vi "Kinect Basic Recorder.vi"() -> ()   [LabVIEW 2011]
uses:
  <vilib>/Utility/sysdir.llb/System Directory Type.ctl
  <vilib>/vision/NI_Vision_Development_Module.lvlib
panel:
  in  "Contour Length Threshold":dbl(slide)=126.92307692307692 min=-32768.0 max=32768.0 step=1.0 scale=0.0..500.0
  in  "Display Type":T1(ring)=enum."Baseline Extracted"
  in  "Post Extraction Limit":cluster{dbl, dbl}(slide)={48.0, 888.0} scale=-3000.0..3000.0
  in  "stop 2":bool
  in  "# Frames in Average":i32=100
  in  "Start":bool
  in  "Zero Out Baseline":bool
  in  "Median Filter Size":i32=5 min=0 max=7
  in  "Divisor":sgl=0.5 min=0 max=1 step=0.1
  in  "Name or Relative Path":string="Mouse Test"
  in  "Distance to Camera Visible":cluster{dbl, dbl}(slide)={-4718.592, 13369.344000000001} scale=-32768.0..32768.0
  in  "Status":string
  out "Frame Display":T2(plugin-control)
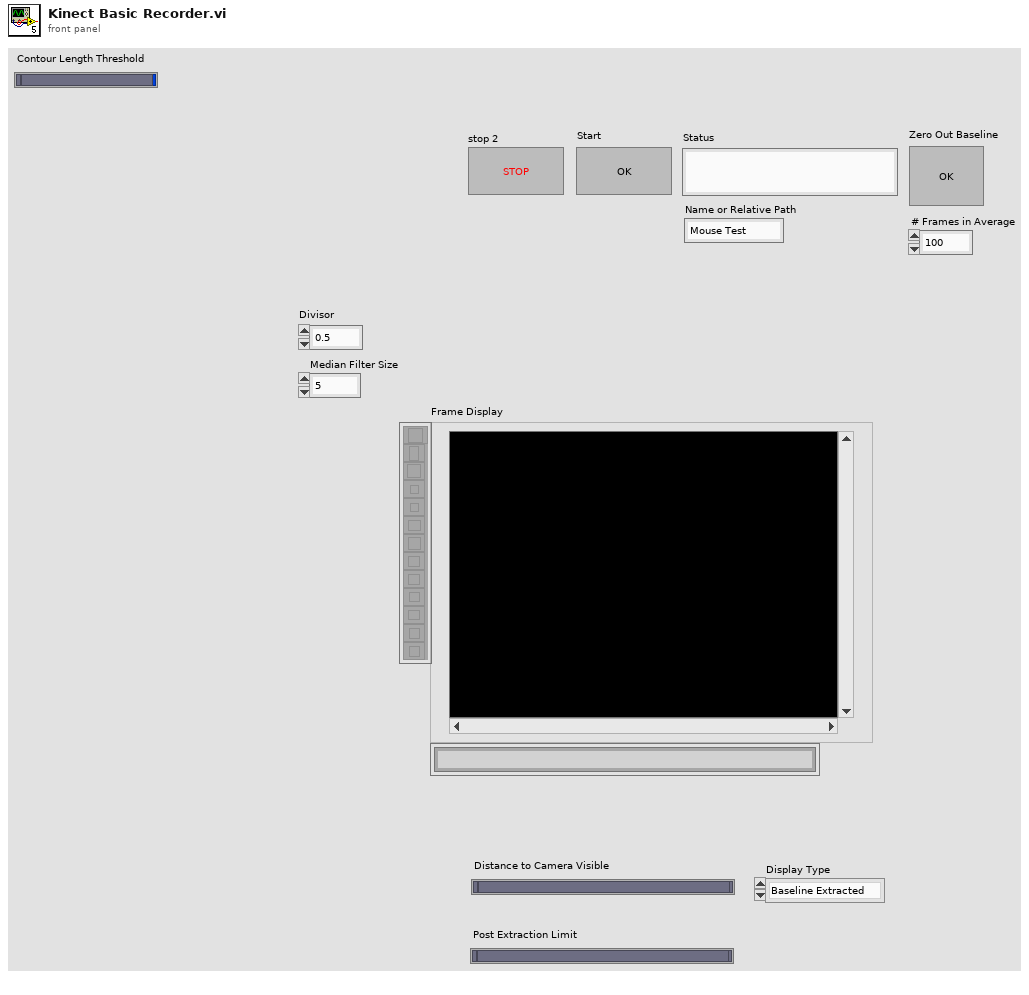
[diagram p1: front panel]
types:
  T1 = enum16{"Raw Image", "Baseline", "Baseline Extracted"}
  T2 = typedef "IMAQ Image.ctl" = refnum<image>
  T3 = typedef "System Directory Type.ctl" = i32
  T4 = enum16{"Record", "Idle", "Acquire Background", "Stop"}
  T5 = enum32{"Average", "Min", "Max", "Clear  if < ", "Clear  if < or =", "Clear  if =", "Clear  if > or =", "Clear  if >"}
  T6 = typedef "Image Type" = u32
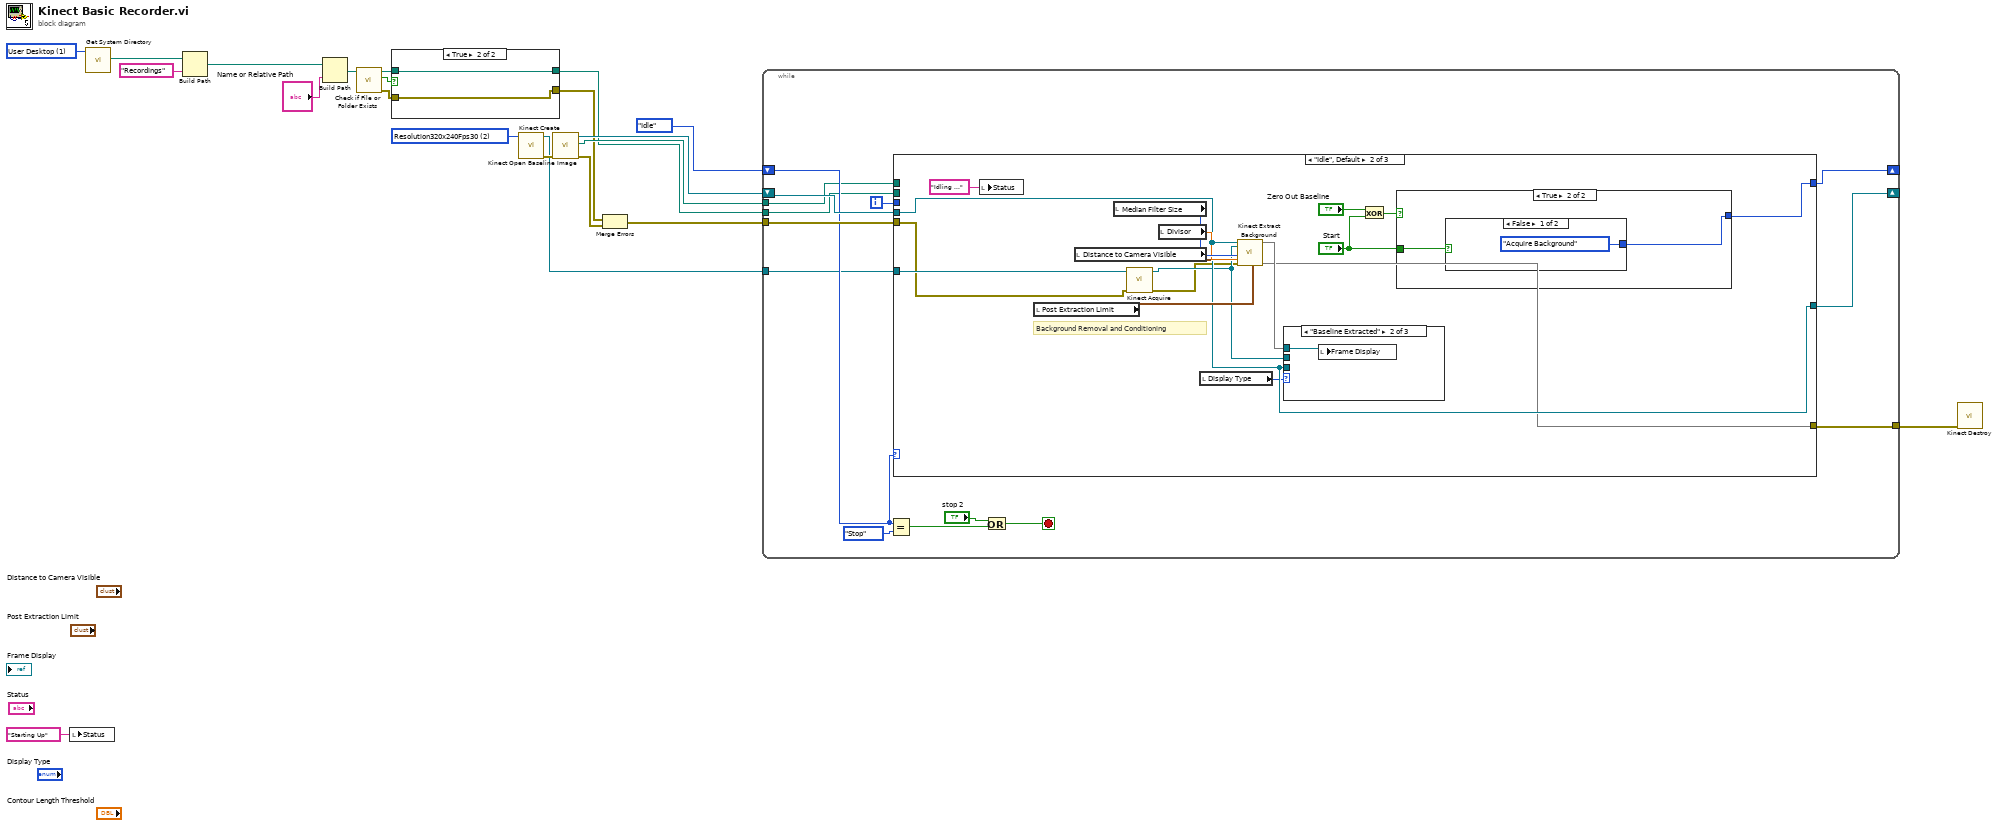
[diagram p0: block diagram]
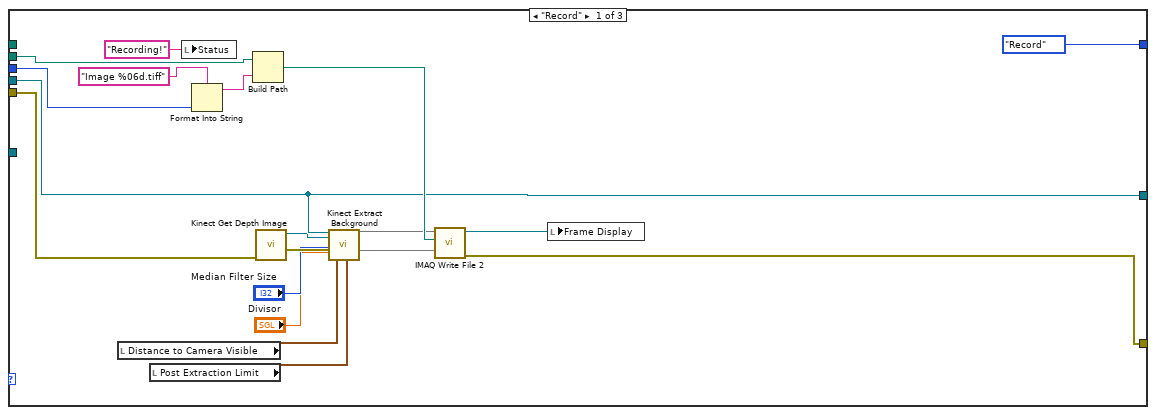
[diagram p2: hidden frame]
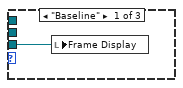
[diagram p3: hidden frame]
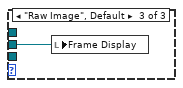
[diagram p4: hidden frame]
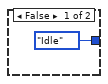
[diagram p5: hidden frame]
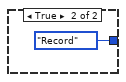
[diagram p6: hidden frame]
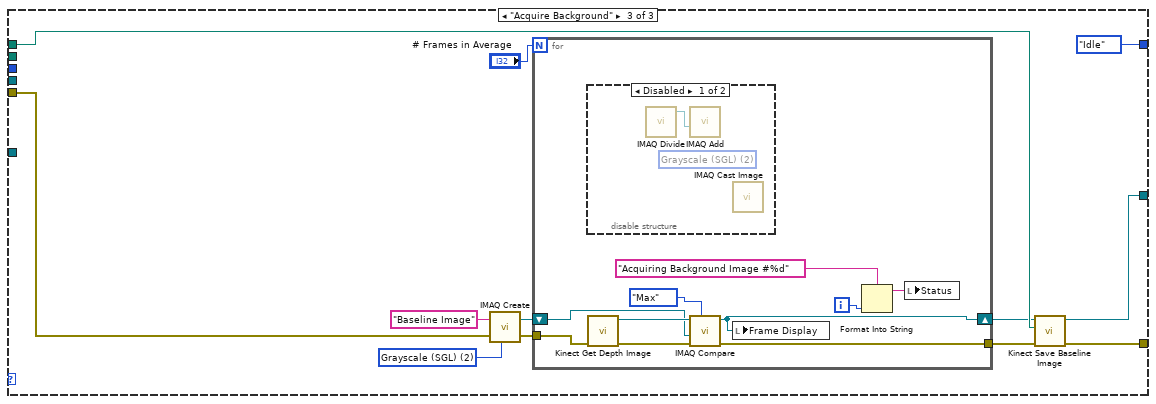
[diagram p7: hidden frame]
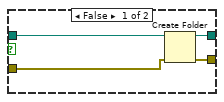
[diagram p9: hidden frame]
diagram:
  w17 = 2 items=["Undefined", "Resolution640x480Fps30", "Resolution320x240Fps30", "Resolution80x60Fps30"] ("Depth Format")
  w19 = T3 1 items=["User Home"=0, "User Desktop"=1, "User Documents"=2, "User Application Data"=3, "User Preferences"=4, "User Temporary"=5, "Public Documents"=6, "Public Application Data"=7, "Public Preferences"=8, "Public Cache"=13, "System Core Libraries"=9, "System Installed Libraries"=10, "Application Files"=11, "Boot Volume Root"=12] ("system directory type")
  n1 = local write "Status"("Starting Up" ("Status")) -> ()
  n2 = call <vilib>:"Get System Directory.vi"("system directory type"=w19) -> ("system directory"=w18:path)  [unwired: 10 in]
  n3 = Build Path(base path=w18, name or relative path="Recordings") -> (appended path=w12:path)
  n4 = Build Path(base path=w12, name or relative path="Name or Relative Path") -> (appended path=w3:path)
  n5 = call <vilib>:"Check if File or Folder Exists.vi"("path"=w3) -> ("error out"=w10:errorcluster, "file or folder exists?"=w8:bool, "dup path"=w9:path)  [unwired: 8 in]
  n6 = case shown="True" w8 {
    tunnel: w10 -> [w25 w26]
    tunnel: w9 -> [w24 w27]
    tunnel: [w22 w27] -> w7
    tunnel: [w23 w26] -> w4
    frame False {
      n7 = Create Folder(path (use dialog)=w24, error in=w25) -> (created path=w22:path, error out=w23:errorcluster)  [unwired: 1 in, 1 out]
    }
    frame True {
    }
  }
  n8 = call "Kinect Create.vi"("Depth Format"=w17) -> ("error out"=w14:errorcluster, "Kinect Acquisition Queue"=w1:refnum<queue>)  [unwired: 9 in]
  n9 = call "Kinect Open Baseline Image.vi"("error in (no error)"=w14) -> ("error out"=w5:errorcluster, "Background Image Path"=w15:path, "Background Image"=w16:T2)  [unwired: 8 in]
  n10 = Merge Errors(w4, w5) -> (w6:errorcluster)
  n11 = while {
    tunnel: w6 -> [w41]
    tunnel: [w40] -> w2
    shift-right: [w33] -> _
    shift-left: T4."Idle" -> [w35]
    shift-right: [w32] -> _
    shift-left: w16 -> [w39]
    tunnel: w15 -> [w31]
    tunnel: w7 -> [w29]
    tunnel: w1 -> [w28]
    i -> [w30]
    stop <- w37 stop-if-true
    n12 = Equal?(x=w35, y=T4."Stop") -> (x = y?=w36:bool)
    n13 = case shown="\"Idle\", Default" w35 {
      tunnel: w41 -> [w53 w62 w93]
      tunnel: [w42 w65 w89] -> w40
      tunnel: w39 -> [w51 w68 _]
      tunnel: [T4."Record" w73 T4."Idle"] -> w33
      tunnel: [w51 w68 w90] -> w32
      tunnel: w31 -> [_ _ w87]
      tunnel: w30 -> [w56 _ _]
      tunnel: w29 -> [w55 _ _]
      tunnel: w28 -> [_ w63 _]
      frame "Record" {
        n14 = local read "Distance to Camera Visible"() -> (w47:cluster{dbl, dbl})
        n15 = local read "Post Extraction Limit"() -> (w46:cluster{dbl, dbl})
        n16 = local write "Status"("Recording!" ("Status")) -> ()
        n17 = Format Into String(format string="Image %06d.tiff", w56) -> (resulting string=w57:string)  [unwired: 2 in, 1 out]
        n18 = Build Path(base path=w55, name or relative path=w57) -> (appended path=w54:path)
        n19 = call "Kinect Get Depth Image.vi"("error in (no error)"=w53) -> ("error out"=w52:errorcluster, "Depth Image"=w50:T2)  [unwired: 9 in]
        n20 = call "Kinect Extract Background.vi"(0:w51, 1:w50, 3:"Median Filter Size", 4:"Divisor", 5:w52, 7:w47, 11:w46) -> (14:w45, 19:w43)  [unwired: 11 in]
        n21 = call-poly "IMAQ Write File 2"("error in (no error)"=w43, "File Path"=w54, "Image"=w45) -> ("error out"=w42:errorcluster, "Image Out (duplicate)"=w44:T2)  [unwired: 7 in]
        n22 = local write "Frame Display"(w44) -> ()
      }
      frame "Idle", Default {
        # "Background Removal and Conditioning"
        n23 = local write "Status"("Idling ..." ("Status")) -> ()
        n24 = local read "Post Extraction Limit"() -> (w69:cluster{dbl, dbl})
        n25 = local read "Distance to Camera Visible"() -> (w70:cluster{dbl, dbl})
        n26 = local read "Median Filter Size"() -> (w72:i32)
        n27 = call "Kinect Acquire.vi"("error in"=w62, "Queue in"=w63) -> ("error out"=w61:errorcluster, "Image Out"=w64:T2)  [unwired: 6 in, 2 out]
        n28 = local read "Divisor"() -> (w71:sgl)
        n29 = local read "Display Type"() -> (w67:T1)
        n30 = call "Kinect Extract Background.vi"(0:w68, 1:w64, 3:w72, 4:w71, 5:w61, 7:w70, 11:w69) -> (14:w66, 19:w65)  [unwired: 11 in]
        n31 = case shown="\"Baseline Extracted\"" w67 {
          tunnel: w66 -> [_ w79 _]
          tunnel: w68 -> [w78 _ _]
          tunnel: w64 -> [_ _ w80]
          frame "Baseline" {
            n32 = local write "Frame Display"(w78) -> ()
          }
          frame "Baseline Extracted" {
            n33 = local write "Frame Display"(w79) -> ()
          }
          frame "Raw Image", Default {
            n34 = local write "Frame Display"(w80) -> ()
          }
        }
        n35 = Exclusive Or(1:"Start", 2:"Zero Out Baseline") -> (0:w75:bool)
        n36 = case shown="True" w75 {
          tunnel: "Start" -> [_ w83]
          tunnel: [T4."Idle" w82] -> w73
          frame False {
          }
          frame True {
            n37 = case shown="False" w83 {
              tunnel: [T4."Acquire Background" T4."Record"] -> w82
              frame False {
              }
              frame True {
              }
            }
          }
        }
      }
      frame "Acquire Background" {
        w96 = T6 2 items=["Grayscale (U8)", "Grayscale (I16)", "Grayscale (SGL)", "Complex (CSG)", "RGB (U32)", "HSL (U32)", "RGB (U64)", "Grayscale (U16)"] ("Image Type")
        n38 = call "IMAQ Create"("Image Name"="Baseline Image", "Image Type"=w96, "error in (no error)"=w93) -> ("New Image"=w95:T2, "error out"=w92:errorcluster)  [unwired: 2 in]
        n39 = for {
          N: "# Frames in Average" -> [_]
          tunnel: w92 -> [w104]
          shift-right: [w98] -> w86
          shift-left: w95 -> [w101]
          tunnel: [w99] -> w88
          i -> [w105]
          n40 = disable-structure shown="Disabled" {
            frame Disabled {
              (unwired) T6 2 items=["Grayscale (U8)", "Grayscale (I16)", "Grayscale (SGL)", "Complex (CSG)", "RGB (U32)", "HSL (U32)", "RGB (U64)", "Grayscale (U16)"] ("Image Type")
              n41 = call "IMAQ Divide"() -> ("Image Dst Out"=w108:T2)  [unwired: 7 in, 1 out]
              n42 = call "IMAQ Add"("Image Src B"=w108) -> ()  [unwired: 6 in, 2 out]
              n43 = call "IMAQ Cast Image"() -> ()  [unwired: 10 in, 2 out]
            }
            frame Enabled {
            }
          }
          n44 = call "Kinect Get Depth Image.vi"("error in (no error)"=w104) -> ("error out"=w100:errorcluster, "Depth Image"=w102:T2)  [unwired: 9 in]
          n45 = call "IMAQ Compare"("Operator"=T5."Max", "error in (no error)"=w100, "Image Src B"=w101, "Image Src A"=w102) -> ("error out"=w99:errorcluster, "Image Dst Out"=w98:T2)  [unwired: 6 in]
          n46 = local write "Frame Display"(w98) -> ()
          n47 = Format Into String(format string="Acquiring Background Image #%d" ("Status"), w105) -> (resulting string=w107:string)  [unwired: 2 in, 1 out]
          n48 = local write "Status"(w107) -> ()
        }
        n49 = call "Kinect Save Baseline Image.vi"("error in (no error)"=w88, "Baseline Image Path"=w87, "Baseline Image"=w86) -> ("error out"=w89:errorcluster, "Baseline Image Out"=w90:T2)  [unwired: 7 in]
      }
    }
    n50 = Or(x="stop 2", y=w36) -> (x .or. y?=w37:bool)
  }
  n51 = call "Kinect Destroy.vi"("error in"=w2) -> ()  [unwired: 10 in, 1 out]
